vi "Execute.vi"(8 "error in (no error)":errorcluster, 10 "Context in":refnum<class "Context.lvclass">, 11 "Shutdown Command in":refnum<class "Shutdown Command.lvclass">) -> (0 "error out":errorcluster, 2 "Context out":refnum<class "Context.lvclass">, 3 "Shutdown Command out":refnum<class "Shutdown Command.lvclass">)   [LabVIEW 2016, in "Shutdown Command.lvclass"]
uses:
  Shutdown Command.lvclass
  Context/Context.lvclass
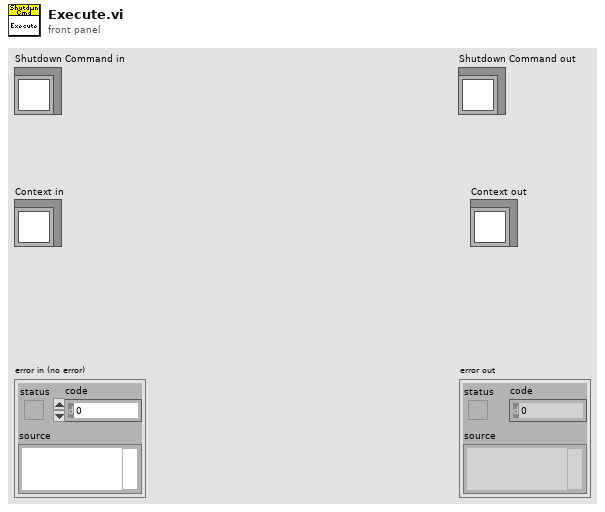
[diagram p1: front panel]
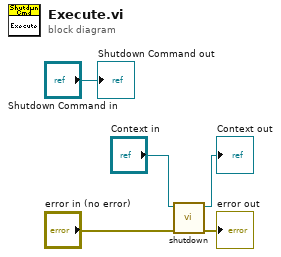
[diagram p0: block diagram]
diagram:
  n1 = call "shutdown.vi"("error in (no error)"="error in (no error)", "Context in"="Context in") -> ("error out"=→"error out":errorcluster, "Context out"=→"Context out":refnum<class "Context.lvclass">)  [unwired: 8 in]
  "Shutdown Command out" <- "Shutdown Command in"
